vi "skip_latter.vi"() -> ()   [LabVIEW 2020]
panel:
  in  "skip_latter":string
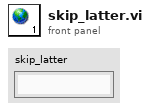
[diagram p1: front panel]
diagram:
